vi "Retrieve_ITX.vi"(0 "File or Folder Path":path=path "F:/Data/SA02703M.20150413/1C - test IV curves/SA02703M.20150413.000100.itx", 5 "offset":i32, 7 "length":i32=1, 9 "index":T2={"A"=3, "B"=4, "C"=2, "D"=4, "E"=3, "N1"=2, "N2"=2, "N3"=3, "N4"=4, "A 1"=9, "A 2"=6, "C 1"=5, "C 2"=1, "E 2"=4}, 11 "stop":bool=TRUE, 12 "file contains 2D data?":bool) -> (1 "Spherical coordinates":dbl[][](array[numeric])=[[0.00040017865219944924, 0.0, 0.0]], 2 "long":cluster{dbl[], dbl[]}(graph)={[0.0], [110244.77019737322]}, 3 "Hall":cluster{dbl[], dbl[]}(graph), 4 "A vs B":cluster{dbl[], dbl[]}[](graph), 6 "C vs D":cluster{dbl[], dbl[]}[](graph), 8 "E( = A)":dbl[][](graph)=[[110378.68665774087], [110980.07953423278], [111495.19477360715], [111915.64471406843], [112233.04169382133], [112438.99805107038], [112525.12612402013], [112470.16366997639], [112217.68994206947], [111789.70029438953], [111274.23469387495], [110766.69750500542], [110316.97859646789], [109965.90599441835], [109773.92869714265], [109789.787277416], [110003.75397996473], [110363.20178239152], [110825.46573983904], [111348.36545048369], [111855.00794926165], [112250.39598352354], [112483.42432276583], [112552.70998905538], [112451.83315132369], [112162.78763826564], [111713.25466935002], [111191.21035273345], [110694.53724896224], [110279.5928782201], [109989.97380978541], [109882.31541094914], [110001.80714213061], [110341.30589836095], [110842.1842343138], [111443.06122538866], [112081.47898242007], [112661.64289264083], [113067.18673431673], [113233.03936114223], [113175.07122823723], [112941.16176104735], [112582.29758727067], [112204.36871268964], [111991.27602015527], [112170.84400908768], [112964.96103502632], [114564.66611351601], [117121.01129687452], [120719.00044431988], [125285.26489471828], [130499.24264731152], [135883.25581660063], [140896.05676770868], [144942.82019698108], [147479.0650178162], [148202.48031258385], [147120.16646143346], [144447.7211176679], [140509.45258195922], [135768.793280923], [130795.33355399042], [126073.75186662724], [121853.2837742944], [118229.44306087599], [115224.2063513687], [112768.31482223286], [110731.56314134419], [108995.87798255129], [107483.6763893677], [106128.78541455646], [104855.46451036901], [103607.3118696334], [102384.2313765957], [101230.33130076929], [100186.07022431206], [99266.21998676342], [98497.26305740117], [97926.34833778953], [97591.55577891736], [97490.47919271766], [97591.9778085518], [97864.74473725742], [98265.71984487999], [98718.65670667142], [99129.3974923125], [99435.6919852036], [99614.92935330104], [99645.7264217609], [99505.59608326468], [99218.37608097591], [98864.30485622029], [98529.85038099214], [98263.54220584434], [98102.40883745131], [98090.42823878347], [98255.61368849514], [98580.8762891815], [99011.32459624425], [99490.59719931691], [99961.62052224239], [100350.2417107682], [100579.03978160745], [100615.02751627413], [100476.70501825697], [100185.46251922955], [99752.95058667203], [99227.61872624676], [98702.74828546104], [98266.72944558918], [97958.96468554964], [97797.5511618173], [97806.86280047648], [97999.64243323806], [98345.7136938256], [98778.07356823028], [99236.5893407795], [99668.38834044256], [100006.21218982217], [100185.94306404449], [100191.80554307303], [100059.23263684074], [99829.25562862752], [99529.86419443425], [99211.7899643557], [98957.91818340262], [98844.62261982085], [98896.14531009043], [99103.43371939835], [99459.99377074702], [99953.85365080244], [100538.34588303909], [101135.71200176232], [101681.3999259956], [102129.91386516251], [102429.60998779481], [102531.40144218317], [102448.58592846889], [102281.52553319387], [102181.61329758061], [102322.36296339578], [102913.49272394249], [104210.42897739566], [106504.34870034066], [110032.59718453824], [114842.91285410528], [120760.15389881792], [127410.28513602099], [134212.2913953614], [140449.95205824668], [145492.10615082897], [148907.71054656434], [150432.79841227608], [149978.72195375955], [147745.39824321677], [144233.99584174476], [140040.09578664508], [135635.47171910867], [131381.10257433544], [127564.99435722757], [124337.61818896537], [121701.36197946641], [119614.84213643732], [118031.00044003755], [116857.95362280619], [115957.65275353614], [115196.23861912514], [114490.8982142473], [113795.16927631399], [113058.96822821294], [112244.72819392942], [111378.94410760995], [110549.0053310049], [109845.67895124746], [109315.01512815294], [108986.52408987831], [108897.85927631223], [109073.84788516775], [109483.51450371224], [110043.79892155928], [110675.0197678782], [111305.59928839048], [111840.76366713356], [112177.79729573772], [112271.55096404631], [112144.47231162751], [111826.34331320488], [111337.0310241983], [110740.64967540494], [110153.23210362448], [109682.00284869647], [109375.08973541405], [109255.38765728302], [109349.5549739555], [109665.51809950397], [110160.07955791596], [110747.46255607209], [111351.56135372884], [111912.19945983191], [112353.14377320139], [112589.91877659422], [112591.2427023089], [112398.88350281748], [112067.99682391841], [111629.24894241171], [111138.87783984812], [110698.25922584705], [110402.3306858104], [110283.88899650435], [110338.47405770053], [110563.57310737768], [110941.29414981174], [111406.78538114014], [111863.96324844705], [112244.83373787144], [112510.18932999922], [112607.97966187482], [112487.23151390854], [112157.43344463283], [111696.00237577481], [111187.33137280052], [110680.87265350664], [110231.66836040841], [109922.32615120923], [109827.16952294615], [109958.96923042976], [110281.70576955267], [110758.57365604518], [111345.46682827664], [111959.57651870661], [112493.11565775092], [112877.35216639875], [113090.14657399816], [113103.852775146], [112886.4488651429], [112464.45015304099], [111932.99484992346], [111390.20775932746], [110892.87547150157], [110502.83300424347], [110301.86923998782], [110340.76068397041], [110587.6815316462], [110943.10993100057], [111288.74092132156], [111493.27130024515], [111408.5459465914], [110878.77087738905], [109756.38601349422], [107810.24000012234], [103835.66849934564], [95185.65881623451], [88446.13043271724], [86867.59351206302], [89503.15683523139], [95095.01600310975], [102549.14145070945], [110873.33829532983], [119094.01322028167], [126194.8528802878], [131072.11021674852], [132429.00219322505], [128875.26455761884], [121093.20873390525], [116526.27832324163], [114840.47424330488], [113966.97892614325], [113507.26059766897], [113310.42757576848], [113260.70006050536], [113263.21679548889], [113241.89726875313], [113152.62411882615], [112966.7328472962], [112655.2522656681], [112209.49642147339], [111670.02075291962], [111116.40574847507], [110612.87560247447], [110203.09644110285], [109945.001841033], [109901.69262242694], [110083.02023719899], [110430.6399368498], [110875.00187728103], [111369.20513018404], [111851.32247972445], [112226.37622050244], [112408.75921671372], [112375.74519629097], [112150.61608586447], [111757.29491710507], [111232.89622869075], [110657.36582605184], [110138.15489960634], [109749.24361185529], [109521.42347160389], [109486.52346882147], [109679.23472886349], [110081.55545782074], [110608.97075945392], [111174.45692967015], [111731.74739813479], [112231.18012024868], [112591.82914004123], [112785.22880849839], [112814.72049475239], [112655.12865287602], [112281.2777369422], [111667.99220102381], [110790.0964991936]], 10 "N":cluster{"N1":dbl, "N2":dbl, "N3":dbl, "N4":dbl}={"N1"=0.0, "N2"=0.0, "N3"=0.00040017865219944924, "N4"=4.737366367530345e-09} {"N4" format="%#_6p"; "N3" format="%#_6p"; "N2" format="%#_6p"; "N1" format="%#_6p"}, 13 "Index, Wavenames":string[][](table)=[["0", "'time.SA02703M.20150413.000100'\n"], ["1", "'temp.SA02703M.20150413.000100'\n"], ["2", "'B.SA02703M.20150413.000100'\n"], ["3", "'Vsource.SA02703M.20150413.000100'\n"], ["4", "'Lockin0.SA02703M.20150413.000100'\n"], ["5", "'Lockin1.SA02703M.20150413.000100'\n"], ["6", "'Lockin2.SA02703M.20150413.000100'\n"], ["7", "'Lockin3.SA02703M.20150413.000100'\n"], ["8", "'Lockin4.SA02703M.20150413.000100'\n"], ["9", "'Lockin5.SA02703M.20150413.000100'\n"], ["10", "'B_rate.SA02703M.20150413.000100'\n"], ["11", "'DC0.SA02703M.20150413.000100'\n"], ["12", "'DC1.SA02703M.20150413.000100'\n"], ["13", "'DC2.SA02703M.20150413.000100'\n"], ["14", "'DC3.SA02703M.20150413.000100'\n"], ["15", "'DC4.SA02703M.20150413.000100'\n"], ["16", "'DC5.SA02703M.20150413.000100'\n"], ["17", "'DC6.SA02703M.20150413.000100'\n"], ["18", "'DC7.SA02703M.20150413.000100'\n"], ["", ""]], 14 "Comments":string="IGOR\nX// Date: 4/13/2015 10:46 PM\nX// SA02703M.20150413\nX// Vbg=0.15V\nX// \nX// B= +0T\nX// Sweep Vsg: 0mV to 100mV, 1mV steps\nX// \nX// lockin\nX// 0: 1, current\nX// 1: 2\nX// 2: 3\nX// 3: 5, \nX// 4: 7, current, 2mV AC, -350uV DC, 0.4 Hz\nX// 5: 9, \nX// appliedVsg= 0.100000\nX// Bx= 0.000000\n\n\n\n\n\n\n\n\n\n\n\n\n\n\n\n\n\n\n\n\n\n\n\n\n\n\n\n\n\n\n\n\n\n\n\n\n\n\n\n\nX \nX Display/R 'time.SA02703M.20150413.000100'\nX AppendToGraph 'temp.SA02703M.20150413.000100'\nX AppendToGraph 'B.SA02703M.20150413.000100'\nX AppendToGraph 'Vsource.SA02703M.20150413.000100'\nX AppendToGraph 'Lockin0.SA02703M.20150413.000100'\nX AppendToGraph 'Lockin1.SA02703M.20150413.000100'\nX AppendToGraph 'Lockin2.SA02703M.20150413.000100'\nX AppendToGraph 'Lockin3.SA02703M.20150413.000100'\nX AppendToGraph 'Lockin4.SA02703M.20150413.000100'\nX AppendToGraph 'Lockin5.SA02703M.20150413.000100'\nX AppendToGraph 'B_rate.SA02703M.20150413.000100'\nX AppendToGraph 'DC0.SA02703M.20150413.000100'\nX AppendToGraph 'DC1.SA02703M.20150413.000100'\nX AppendToGraph 'DC2.SA02703M.20150413.000100'\nX AppendToGraph 'DC3.SA02703M.20150413.000100'\nX AppendToGraph 'DC4.SA02703M.20150413.000100'\nX AppendToGraph 'DC5.SA02703M.20150413.000100'\nX AppendToGraph 'DC6.SA02703M.20150413.000100'\nX AppendToGraph 'DC7.SA02703M.20150413.000100'\nX Label bottom \"x label\"\nX Label left \"y label\"\nX ModifyGraph rgb('time.SA02703M.20150413.000100')=(65280,0,0)\nX ModifyGraph rgb('temp.SA02703M.20150413.000100')=(65280,18432,0)\nX ModifyGraph rgb('B.SA02703M.20150413.000100')=(65280,36864,0)\nX ModifyGraph rgb('Vsource.SA02703M.20150413.000100')=(65280,55296,0)\nX ModifyGraph rgb('Lockin0.SA02703M.20150413.000100')=(57344,65280,0)\nX ModifyGraph rgb('Lockin1.SA02703M.20150413.000100')=(37376,65280,0)\nX ModifyGraph rgb('Lockin2.SA02703M.20150413.000100')=(18944,65280,0)\nX ModifyGraph rgb('Lockin3.SA02703M.20150413.000100')=(512,65280,0)\nX ModifyGraph rgb('Lockin4.SA02703M.20150413.000100')=(0,65280,17920)\nX ModifyGraph rgb('Lockin5.SA02703M.20150413.000100')=(0,65280,36352)\nX ModifyGraph rgb('B_rate.SA02703M.20150413.000100')=(0,65280,54784)\nX ModifyGraph rgb('DC0.SA02703M.20150413.000100')=(0,57856,65280)\nX ModifyGraph rgb('DC1.SA02703M.20150413.000100')=(0,39424,65280)\nX ModifyGraph rgb('DC2.SA02703M.20150413.000100')=(0,20992,65280)\nX ModifyGraph rgb('DC3.SA02703M.20150413.000100')=(0,2560,65280)\nX ModifyGraph rgb('DC4.SA02703M.20150413.000100')=(17408,0,65280)\nX ModifyGraph rgb('DC5.SA02703M.20150413.000100')=(35840,0,65280)\nX ModifyGraph rgb('DC6.SA02703M.20150413.000100')=(54272,0,65280)\nX ModifyGraph rgb('DC7.SA02703M.20150413.000100')=(65280,0,58368)\nX Legend/C/N=text0/J \"\\\\s('time.SA02703M.20150413.000100') time\\r\\\\s('temp.SA02703M.20150413.000100') temp\\r\\\\s('B.SA02703M.20150413.000100') B\\r\\\\s('Vsource.SA02703M.20150413.000100') Vsource\\r\\\\s('Lockin0.SA02703M.20150413.000100') Lockin0\\r\\\\s('Lockin1.SA02703M.20150413.000100') Lockin1\\r\\\\s('Lockin2.SA02703M.20150413.000100') Lockin2\\r\\\\s('Lockin3.SA02703M.20150413.000100') Lockin3\\r\\\\s('Lockin4.SA02703M.20150413.000100') Lockin4\\r\\\\s('Lockin5.SA02703M.20150413.000100') Lockin5\\r\\\\s('B_rate.SA02703M.20150413.000100') B_rate\\r\\\\s('DC0.SA02703M.20150413.000100') DC0\\r\\\\s('DC1.SA02703M.20150413.000100') DC1\\r\\\\s('DC2.SA02703M.20150413.000100') DC2\\r\\\\s('DC3.SA02703M.20150413.000100') DC3\\r\\\\s('DC4.SA02703M.20150413.000100') DC4\\r\\\\s('DC5.SA02703M.20150413.000100') DC5\\r\\\\s('DC6.SA02703M.20150413.000100') DC6\\r\\\\s('DC7.SA02703M.20150413.000100') DC7\"\nX ModifyGraph mirror(bottom)=1\nX ModifyGraph width=216\nX ModifyGraph height={Aspect,0.6}\nX ModifyGraph Log(bottom)=0\nX ModifyGraph Log(left)=0\nX \n", 15 "E index vs Field":cluster{dbl[], dbl[]}(graph)={[0.0], [110378.68665774087]})   [LabVIEW 2013]
uses:
  <vilib>/Utility/miscctls.llb/LVOffsetAndMultiplierTypeDef.ctl
  <vilib>/Analysis/2dsp.llb/Decimate (single shot, DBL).vi
  <vilib>/Analysis/3filter.llb/Savitzky-Golay Filter (DBL).vi
  <vilib>/Analysis/NI_AALPro.lvlib
  <vilib>/Analysis/NI_AALBase.lvlib
panel:
  in  "VRM mode":bool
  in  "Ring":u16(ring) items=["default", "DIFF"]
  in  "decimating factor":i32=1
  in  "decimate files":i32=1
  in  "side points":i32=6
  in  "fit points":dbl=10.0
  in  "dy/dx vs x":bool=TRUE
  in  "Portion of data":cluster{dbl, dbl}(slide)={0.75, 0.25} scale=0.0..1.0
  in  "length 2":i32=1000
  in  "index 2":i32
  out "Ns":T1(array[cluster])=[{"N1"=0.0, "N2"=0.0, "N3"=0.00040017865219944924, "N4"=4.737366367530345e-09}]
  in  "SE?":bool
  in  "D  is time?":bool
  in  "B is time?":bool
  out "time":string[][](table)=[["4/13/2015", "10:46 PM"]]
  in  "Use Folder Index File?":bool
  in  "Generate Folder Index File?":bool
  in  "Ez name":string="Conductance (S)"
  in  "Ey name":string="BY (T)"
  in  "Ex name":string="Vsg (mV)"
  in  "C y name":string="C y name"
  in  "D x name":string="D x name"
  in  "A y name":string="4Term R (Ohm)"
  in  "B x name":string="time"
  in  "recolor traces?":bool
  in  "Ex":T3={"Offset"=0.0, "Multiplier"=1.0}
  in  "Ey":T3={"Offset"=0.0, "Multiplier"=1.0}
  out "Path":path=path "F:/Data/SA02703M.20150413/1C - test IV curves/SA02703M.20150413.000100.itx"
  out "counter":i32
  in  "pattern":string="*.itx"
  # "A1-A2\nC1-C2\nE-E2"
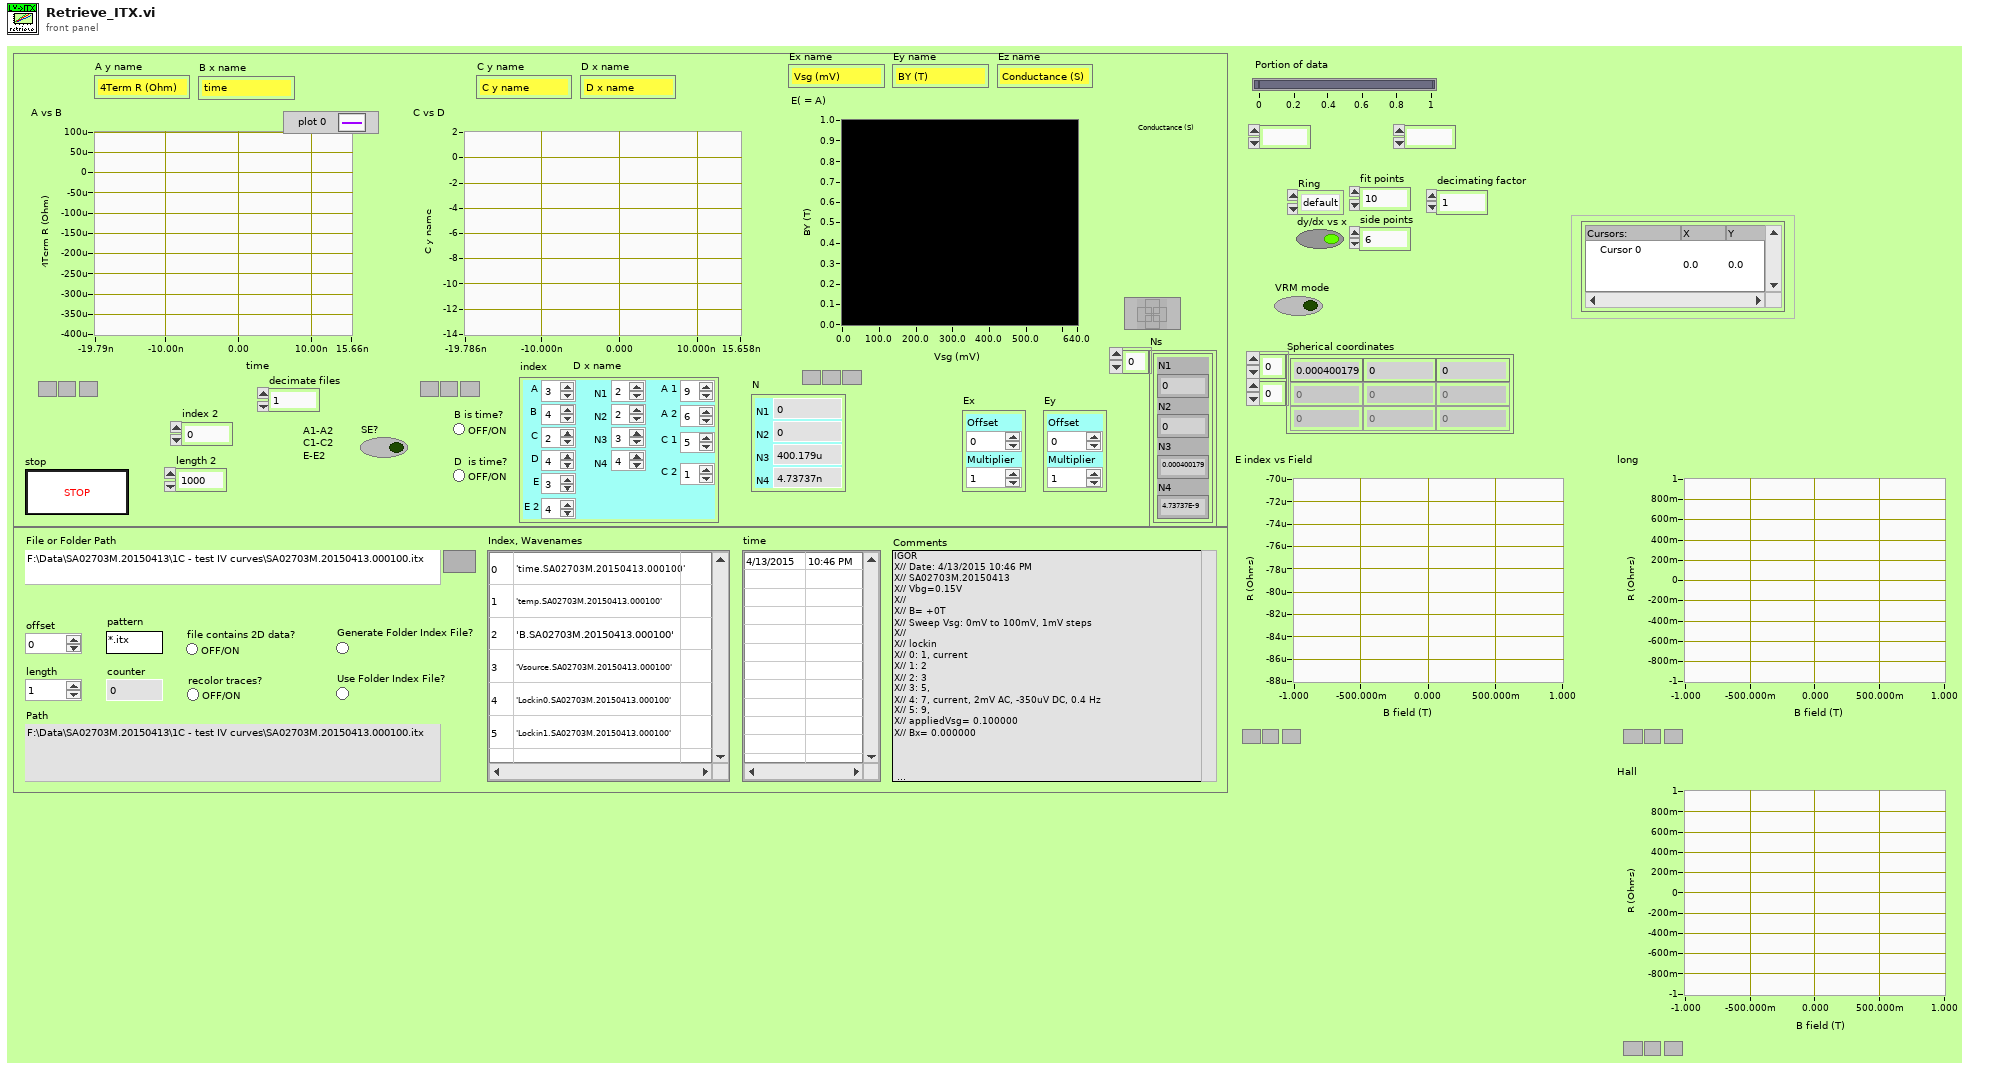
[diagram p1: front panel]
types:
  T1 = cluster{"N1":dbl, "N2":dbl, "N3":dbl, "N4":dbl}[]
  T2 = cluster{"A":i32, "B":i32, "C":i32, "D":i32, "E":i32, "N1":i32, "N2":i32, "N3":i32, "N4":i32, "A 1":i32, "A 2":i32, "C 1":i32, "C 2":i32, "E 2":i32}
  T3 = typedef "LVOffsetAndMultiplierTypeDef.ctl" = cluster{"Offset":dbl, "Multiplier":dbl}
  T4 = cluster{"Decimated Array":dbl[], "Decimated Array":dbl[]}
  T5 = cluster{"Decimated Array":dbl[], "Filtered X":dbl[]}
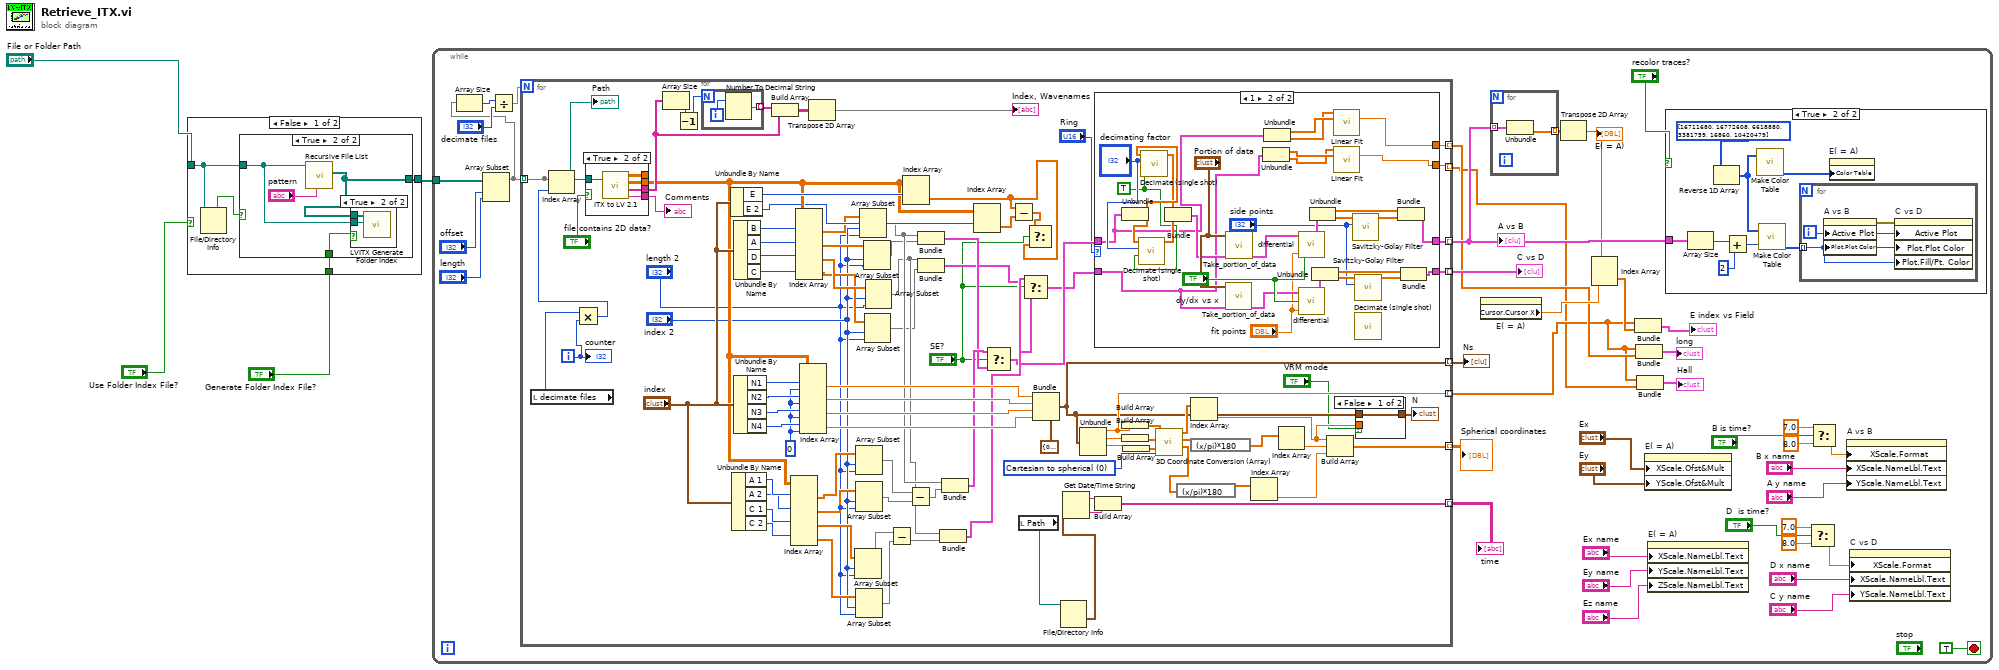
[diagram p0: block diagram]
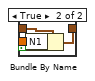
[diagram p3: hidden frame]
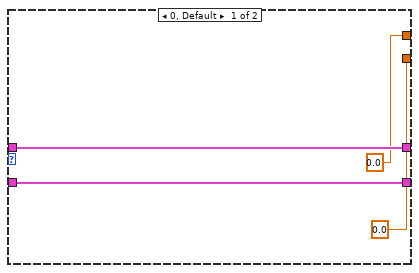
[diagram p4: hidden frame]
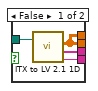
[diagram p5: hidden frame]
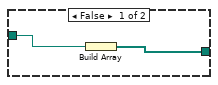
[diagram p6: hidden frame]
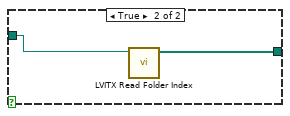
[diagram p8: hidden frame]
diagram:
  n1 = case shown="False" "Use Folder Index File?" {
    tunnel: [w6 w17] -> w2
    tunnel: "File or Folder Path" -> [w8 w18]
    tunnel: "Generate Folder Index File?" -> [w5 _]
    frame False {
      n2 = File/Directory Info(path=w8) -> (directory=w7:bool)  [unwired: 1 in, 6 out]
      n3 = case shown="True" w7 {
        tunnel: [w10 w13] -> w6
        tunnel: w8 -> [w9 w12]
        tunnel: w5 -> [_ w11]
        frame False {
          n4 = Build Array(w9) -> (w10:path[])
        }
        frame True {
          n5 = call <vilib>:"Recursive File List.vi"("pattern"="pattern", "Folder Path"=w12) -> ("All Files in Dir"=w13:path[])  [unwired: 5 in, 4 out]
          n6 = case shown="True" w11 {
            tunnel: w13 -> [_ w16]
            tunnel: w12 -> [_ w15]
            frame False {
            }
            frame True {
              n7 = call <userlib>:"LVITX Generate Folder Index.vi"("File or Folder Path"=w15, "All Files in Dir"=w16) -> ()  [unwired: 10 in]
            }
          }
        }
      }
    }
    frame True {
      n8 = call <userlib>:"LVITX Read Folder Index.vi"("File or Folder Path"=w18) -> ("Array"=w17:path[])  [unwired: 10 in]
    }
  }
  n9 = while {
    tunnel: w2 -> [w33]
    stop <- TRUE stop-if-true
    n10 = Array Subset(array=w33, index="offset", length="length") -> (w29:path[])
    n11 = Array Size(array=w29) -> (size(s)=w32:i32)
    n12 = Divide(x=w32, y="decimate files") -> (x/y=w30:dbl)
    n13 = for {
      N: w30 -> [_]
      tunnel: w29 -> [w165]
      tunnel: [w165] -> _ mode=indexing
      tunnel: [w88] -> w36 mode=indexing
      tunnel: [w87] -> w56 mode=indexing
      tunnel: [w139] -> w48 mode=indexing
      tunnel: [w75] -> w37 mode=indexing
      tunnel: [w86] -> w34 mode=indexing
      tunnel: [w81] -> w21 mode=indexing
      tunnel: [w79] -> w24 mode=indexing
      tunnel: [w78] -> w20 mode=indexing
      i -> [w84]
      w103 = u16 0 items=["Cartesian to spherical", "spherical to Cartesian", "Cartesian to cylindrical", "cylindrical to Cartesian", "spherical to cylindrical", "cylindrical to spherical"] ("conversion type")
      w137 = 0 ("disabled index (col)")
      n14 = local read "decimate files"() -> (w82:i32)
      n15 = Multiply(x=w82, y=w84) -> (x*y=w83:i32)
      n16 = Index Array(array=w165, index=w83) -> (element=w85:path)
      "Path" <- w85
      n17 = case shown="True" "file contains 2D data?" {
        tunnel: [w211 w214] -> w166
        tunnel: [w209 w215] -> w125
        tunnel: w85 -> [w210 w216]
        tunnel: [w208 w213] -> w158
        tunnel: [w209 w212] -> _
        frame False {
          n18 = call <userlib>:"ITX to LV 2.1 1D.vi"("file (use dialog)"=w210) -> ("1D arrays"=w209:dbl[][], "wave names"=w208:string[], "Notes"=w211:string)  [unwired: 2 in]
        }
        frame True {
          n19 = call <userlib>:"ITX to LV 2.1.vi"("file (use dialog)"=w216) -> ("2D array"=w212:dbl[][], "1D arrays"=w215:dbl[][], "wave names"=w213:string[], "Notes"=w214:string)  [unwired: 1 in]
        }
      }
      "Comments" <- w166
      n20 = Array Size(array=w158) -> (size(s)=w161:i32)
      n21 = Decrement(x=w161) -> (x-1=w160:i32)
      n22 = for {
        N: w160 -> [_]
        tunnel: [w206] -> w163 mode=indexing
        i -> [w207]
        n23 = Number To Decimal String(number=w207) -> (decimal integer string=w206:string)  [unwired: 1 in]
      }
      n24 = Unbundle By Name("index") -> ("E"=w151:i32, "E 2"=w124:i32)
      n25 = Unbundle By Name("index") -> ("A 1"=w136:i32, "A 2"=w135:i32, "C 1"=w134:i32, "C 2"=w133:i32)
      n26 = Unbundle By Name("index") -> ("B"=w150:i32, "A"=w149:i32, "D"=w148:i32, "C"=w147:i32)
      n27 = Unbundle By Name("index") -> ("N1"=w152:i32, "N2"=w153:i32, "N3"=w154:i32, "N4"=w155:i32)
      n28 = Build Array(w163, w158) -> (w159:string[][])
      n29 = Index Array(array=w125, index (row) #1=w136, index (row) #2=w135, index (row) #3=w134, index (row) #4=w133) -> (element #1=w112:dbl[], element #2=w110:dbl[], element #3=w109:dbl[], element #4=w107:dbl[])  [unwired: 4 in]
      n30 = Index Array(array=w125, index (row) #1=w150, index (row) #2=w149, index (row) #3=w148, index (row) #4=w147) -> (element #1=w120:dbl[], element #2=w118:dbl[], element #3=w116:dbl[], element #4=w114:dbl[])  [unwired: 4 in]
      n31 = Index Array(array=w125, index (row) #1=w152, index (col) #1=w137, index (row) #2=w153, index (col) #2=w137, index (row) #3=w154, index (col) #3=w137, index (row) #4=w155, index (col) #4=w137) -> (element #1=w143:dbl, element #2=w144:dbl, element #3=w145:dbl, element #4=w157:dbl)
      n32 = Transpose 2D Array(2D array=w159) -> (transposed array=→"Index, Wavenames":string[][])
      n33 = Array Subset(array=w109, index="index 2", length="length 2") -> (w108:dbl[])
      n34 = Array Subset(array=w112, index="index 2", length="length 2") -> (w111:dbl[])
      n35 = Array Subset(array=w110, index="index 2", length="length 2") -> (w77:dbl[])
      n36 = Array Subset(array=w107, index="index 2", length="length 2") -> (w106:dbl[])
      n37 = Array Subset(array=w120, index="index 2", length="length 2") -> (w119:dbl[])
      n38 = Array Subset(array=w118, index="index 2", length="length 2") -> (w117:dbl[])
      n39 = Array Subset(array=w114, index="index 2", length="length 2") -> (w113:dbl[])
      n40 = Array Subset(array=w116, index="index 2", length="length 2") -> (w115:dbl[])
      n41 = Subtract(x=w108, y=w106) -> (x-y=w131:dbl[])
      n42 = Index Array(array=w125, index (row)=w151) -> (element=w123:dbl[])  [unwired: 1 in]
      n43 = Subtract(x=w111, y=w77) -> (x-y=w132:dbl[])
      n44 = Bundle(w119, w117) -> (w128:cluster{dbl[], dbl[]})  [unwired: 1 in]
      n45 = Bundle(w115, w113) -> (w127:cluster{dbl[], dbl[]})  [unwired: 1 in]
      n46 = Bundle(w115, w131) -> (w129:cluster{dbl[], dbl[]})  [unwired: 1 in]
      n47 = Bundle(w119, w132) -> (w130:cluster{dbl[], dbl[]})  [unwired: 1 in]
      n48 = Index Array(array=w125, index (row)=w124) -> (element=w122:dbl[])  [unwired: 1 in]
      n49 = Select(t=w130, s="SE?", f=w128) -> (s? t:f=w90:cluster{dbl[], dbl[]})
      n50 = Subtract(x=w123, y=w122) -> (x-y=w121:dbl[])
      n51 = local read "Path"() -> (w146:path)
      n52 = Select(t=w129, s="SE?", f=w127) -> (s? t:f=w89:cluster{dbl[], dbl[]})
      n53 = Select(t=w121, s="SE?", f=w123) -> ()  [unwired: 1 out]
      n54 = Bundle(cluster=cluster{"N1":dbl, "N2":dbl, "N3":dbl, "N4":dbl} {"N1"=0.0, "N2"=0.0, "N3"=0.0, "N4"=0.0}, "N1"=w143, "N2"=w144, "N3"=w145, "N4"=w157) -> (w75:cluster{"N1":dbl, "N2":dbl, "N3":dbl, "N4":dbl})
      n55 = File/Directory Info(path=w146) -> (last mod=w142:timestamp)  [unwired: 1 in, 6 out]
      n56 = Get Date/Time String(seconds (now)=w142) -> (date string=w141:string, time string=w140:string)  [unwired: 2 in]
      n57 = Unbundle(w75) -> ("N1"=w81:dbl, "N2"=w102:dbl, "N3"=w99:dbl)  [unwired: 1 out]
      n58 = case shown="1" "Ring" {
        tunnel: w90 -> [w174 w182]
        tunnel: w89 -> [w173 w181]
        tunnel: [w174 w196] -> w88
        tunnel: [w173 w191] -> w87
        tunnel: [0.0 w176] -> w79
        tunnel: [0.0 w175] -> w78
        frame 0, Default {
        }
        frame 1 {
          w183 = TRUE ("averaging")
          n59 = Unbundle(w182) -> (w188:dbl[], w186:dbl[])
          n60 = call-poly <vilib>:"Decimate (single shot).vi"("averaging"=w183, "decimating factor"="decimating factor", "X"=w186) -> ("Decimated Array"=w185:dbl[])  [unwired: 7 in, 1 out]
          n61 = call-poly <vilib>:"Decimate (single shot).vi"("averaging"=w183, "decimating factor"="decimating factor", "X"=w188) -> ("Decimated Array"=w187:dbl[])  [unwired: 7 in, 1 out]
          n62 = Bundle("Decimated Array"=w187, "Decimated Array"=w185) -> (w189:T4)  [unwired: 1 in]
          n63 = call <userlib>:"Take_portion_of_data.vi"("input IV"=w181, "Slide"="Portion of data") -> ("Output IV"=w203:cluster{dbl[], dbl[]})  [unwired: 5 in]
          n64 = call <userlib>:"Take_portion_of_data.vi"("input IV"=w189, "Slide"="Portion of data") -> ("Output IV"=w202:cluster{dbl[], dbl[]})  [unwired: 5 in]
          n65 = Unbundle(w181) -> (w178:dbl[], w177:dbl[])
          n66 = Unbundle(w182) -> (w180:dbl[], w179:dbl[])
          n67 = call <userlib>:"differential.vi"("Numeric"="fit points", "dy/dx vs x"="dy/dx vs x", "A vs B 2"=w202) -> ("A vs B 3"=w197:T4)  [unwired: 1 in]
          n68 = call <userlib>:"differential.vi"("Numeric"="fit points", "dy/dx vs x"="dy/dx vs x", "A vs B 2"=w203) -> ("A vs B 3"=w192:T4)  [unwired: 1 in]
          n69 = Unbundle(w197) -> ("Decimated Array"=w200:dbl[], "Decimated Array"=w198:dbl[])
          n70 = Unbundle(w192) -> ("Decimated Array"=w193:dbl[], "Decimated Array"=w195:dbl[])
          n71 = call <vilib>:"Linear Fit.vi"("Y"=w179, "X"=w180) -> ("slope"=w176:dbl)  [unwired: 9 in, 4 out]
          n72 = call <vilib>:"Linear Fit.vi"("Y"=w177, "X"=w178) -> ("slope"=w175:dbl)  [unwired: 9 in, 4 out]
          n73 = call-poly <vilib>:"Savitzky-Golay Filter.vi"("side points"="side points", "X"=w198) -> ("Filtered X"=w199:dbl[])  [unwired: 8 in, 1 out]
          n74 = call-poly <vilib>:"Savitzky-Golay Filter.vi"("side points"="side points", "X"=w195) -> ("Filtered X"=w194:dbl[])  [unwired: 8 in, 1 out]
          n75 = call-poly <vilib>:"Decimate (single shot).vi"() -> ()  [unwired: 10 in, 2 out]
          n76 = Bundle("Decimated Array"=w200, "Filtered X"=w199) -> (w196:T5)  [unwired: 1 in]
          n77 = Bundle("Decimated Array"=w193, "Filtered X"=w194) -> (w191:T5)  [unwired: 1 in]
        }
      }
      n78 = Build Array(w141, w140) -> (w139:string[])
      n79 = Build Array(w81) -> (w101:dbl[])
      n80 = Build Array(w102) -> (w100:dbl[])
      n81 = Build Array(w99) -> (w98:dbl[])
      n82 = call <vilib>:"3D Coordinate Conversion (Array).vi"("conversion type"=w103, "Axis 3"=w98, "Axis 2"=w100, "Axis 1"=w101) -> ("Axis 3 Out"=w96:dbl[], "Axis 2 Out"=w97:dbl[], "Axis 1 Out"=w95:dbl[])  [unwired: 4 in, 1 out]
      n83 = expression code="(x/pi)*180" ("degrees to radians")(w96) -> (w93:dbl[])
      n84 = Index Array(array=w95) -> (element=w76:dbl)  [unwired: 1 in]
      n85 = expression code="(x/pi)*180" ("degrees to radians")(w97) -> (w94:dbl[])
      n86 = Index Array(array=w93) -> (element=w91:dbl)  [unwired: 1 in]
      n87 = Index Array(array=w94) -> (element=w92:dbl)  [unwired: 1 in]
      n88 = Build Array(w76, w92, w91) -> (w86:dbl[])
      n89 = case shown="False" "VRM mode" {
        tunnel: w76 -> [_ w170]
        tunnel: w75 -> [w167 w169]
        tunnel: [w167 w168] -> w74
        frame False {
        }
        frame True {
          n90 = Bundle By Name(cluster=w169, "N1"=w170) -> (w168:cluster{"N1":dbl, "N2":dbl, "N3":dbl, "N4":dbl})
        }
      }
      "N" <- w74
      "counter" <- w84
    }
    "time" <- w48
    "Ns" <- w37
    "Spherical coordinates" <- w34
    "A vs B" <- w36
    "C vs D" <- w56
    n91 = property on="E( = A)" class="IntGraph (strict)"() -> ("Cursor.Cursor X"=w25:dbl)  [unwired: 2 in, 2 out]
    n92 = for {
      tunnel: w36 -> [w61] mode=indexing
      tunnel: [w60] -> w35 mode=indexing
      n93 = Unbundle(w61) -> ("Filtered X"=w60:dbl[])  [unwired: 1 out]
    }
    n94 = Transpose 2D Array(2D array=w35) -> (transposed array=w28:dbl[][])
    "E( = A)" <- w28
    n95 = Index Array(array=w28, index (row)=w25) -> (element=w27:dbl[])  [unwired: 1 in]
    n96 = Bundle(w21, w27) -> (→"E index vs Field":cluster{dbl[], dbl[]})  [unwired: 1 in]
    n97 = Bundle(w21, w24) -> (→"long":cluster{dbl[], dbl[]})  [unwired: 1 in]
    n98 = Bundle(w21, w20) -> (→"Hall":cluster{dbl[], dbl[]})  [unwired: 1 in]
    n99 = property on="E( = A)" class="IntGraph (strict)"("XScale.Ofst&Mult"="Ex", "YScale.Ofst&Mult"="Ey") -> ()  [unwired: 2 in, 2 out]
    n100 = property on="E( = A)" class="IntGraph (strict)"("XScale.NameLbl.Text"="Ex name", "YScale.NameLbl.Text"="Ey name", "ZScale.NameLbl.Text"="Ez name") -> ()  [unwired: 2 in, 2 out]
    n101 = case shown="True" "recolor traces?" {
      tunnel: w36 -> [_ w64]
      frame False {
      }
      frame True {
        n102 = Array Size(array=w64) -> (size(s)=w65:i32)
        n103 = Reverse 1D Array(array=u32[] [16711680, 16772608, 6618880, 3381759, 16860, 10420479] ("color scale")) -> (reversed array=w63:u32[])
        n104 = Add(x=w65, y=2 ("x")) -> (x+y=w69:i32)
        n105 = call <userlib>:"Make Color Table.vi"("Array"=w63) -> ("Color Tbl"=w67:u32[])  [unwired: 1 in, 3 out]
        n106 = call <userlib>:"Make Color Table.vi"("Array"=w63, "Size/3"=w69) -> ("Color Tbl"=w66:u32[])  [unwired: 3 out]
        n107 = for {
          tunnel: w66 -> [w70] mode=indexing
          i -> [w71]
          n108 = property on="A vs B" class="XYGraph (strict)"("Active Plot"=w71, "Plot.Plot Color"=w70) -> (error out=w72:errorcluster)  [unwired: 2 in, 1 out]
          n109 = property on="C vs D" class="XYGraph (strict)"(error in=w72, "Active Plot"=w71, "Plot.Plot Color"=w70, "Plot.Fill/Pt. Color"=w70) -> ()  [unwired: 1 in, 2 out]
        }
        n110 = property on="E( = A)" class="IntGraph (strict)"("Color Table"=w67) -> ()  [unwired: 2 in, 2 out]
      }
    }
    n111 = Select(t=7.0, s="D  is time?", f=8.0) -> (s? t:f=w42:dbl)
    n112 = Select(t=7.0, s="B is time?", f=8.0) -> (s? t:f=w43:dbl)
    n113 = property on="A vs B" class="XYGraph (strict)"("XScale.Format"=w43, "XScale.NameLbl.Text"="B x name", "YScale.NameLbl.Text"="A y name") -> ()  [unwired: 2 in, 2 out]
    n114 = property on="C vs D" class="XYGraph (strict)"("XScale.Format"=w42, "XScale.NameLbl.Text"="D x name", "YScale.NameLbl.Text"="C y name") -> ()  [unwired: 2 in, 2 out]
  }
